vi "Handle Messages.vi"(8 "error in (no error)":errorcluster, 9 "Message Data":variant, 10 "Message":string, 11 "Mock Rig Process In":refnum<class "Mock Error Handler.lvclass">) -> (0 "error out":errorcluster, 3 "Mock Rig Process Out":refnum<class "Mock Error Handler.lvclass">)   [LabVIEW 2020, in "Mock Error Handler.lvclass"]
uses:
  Mock Error Handler.lvclass
  C:/Users/anton/Documents/GitHub/Triarc-Framework/source/Framework/Process/Process.lvclass
  Mock Error Handler.lvclass/Mock Error Handler.ctl
  Framework/Process/Process.lvclass/Process.ctl
  Framework/Process/Process.lvclass
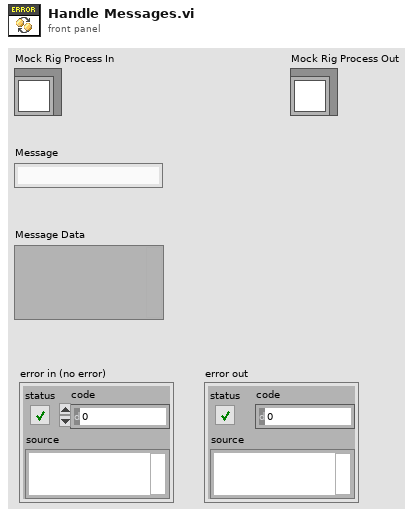
[diagram p1: front panel]
types:
  T1 = cluster{"Message":string, "Message Data":variant}
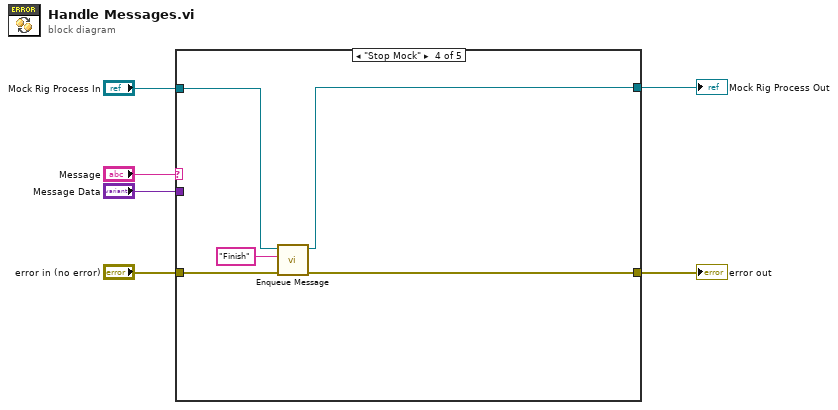
[diagram p0: block diagram]
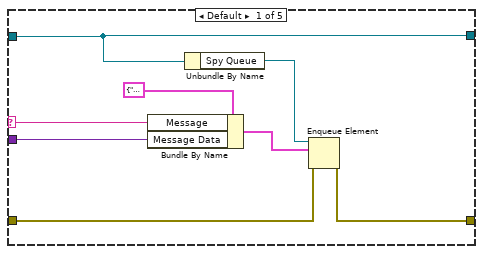
[diagram p2: hidden frame]
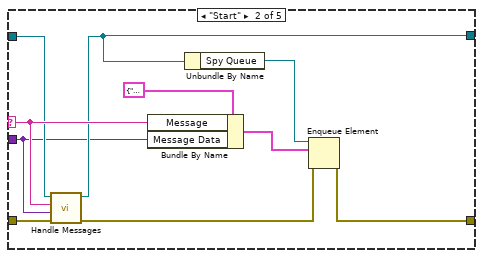
[diagram p3: hidden frame]
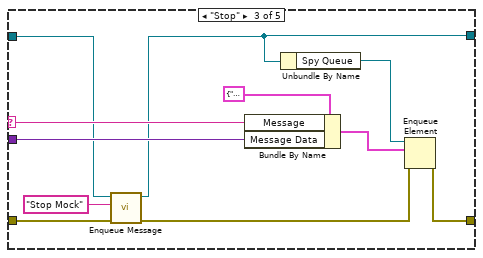
[diagram p4: hidden frame]
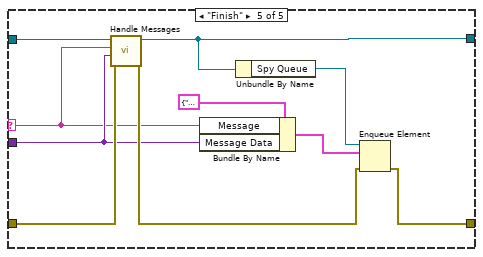
[diagram p5: hidden frame]
diagram:
  n1 = case shown="\"Stop Mock\"" "Message" {
    selector: "Message" -> [w10 w18 w31 _ w41]
    tunnel: [w8 w20 w30 w39 w43] -> w6
    tunnel: [w7 w17 w26 w37 w45] -> w5
    tunnel: "error in (no error)" -> [w9 w21 w27 w38 w49]
    tunnel: "Message Data" -> [w11 w15 w32 _ w42]
    tunnel: "Mock Rig Process In" -> [w7 w16 w25 w36 w50]
    frame Default {
      n2 = Bundle By Name(cluster=T1 {"Message"="", "Message Data"=variant} ("Message Cluster"), "Message"=w10, "Message Data"=w11) -> (w14:T1)
      n3 = Unbundle By Name(w7) -> ("Spy Queue"=w12:refnum<queue>)
      n4 = Enqueue Element(queue=w12, element=w14, error in (no error)=w9) -> (error out=w8:errorcluster)  [unwired: 1 in, 2 out]
    }
    frame "Start" {
      n5 = call-parent "Handle Messages.vi"("error in (no error)"=w21, "Message Data"=w15, "Message"=w18, "Process In"=w16) -> ("error out"=w19:errorcluster, "Process Out"=w17:refnum<class "Mock Error Handler.lvclass">)  [unwired: 6 in]
      n6 = Bundle By Name(cluster=T1 {"Message"="", "Message Data"=variant} ("Message Cluster"), "Message"=w18, "Message Data"=w15) -> (w24:T1)
      n7 = Unbundle By Name(w17) -> ("Spy Queue"=w22:refnum<queue>)
      n8 = Enqueue Element(queue=w22, element=w24, error in (no error)=w19) -> (error out=w20:errorcluster)  [unwired: 1 in, 2 out]
    }
    frame "Stop" {
      n9 = call "Enqueue Message.vi"("error in (no error)"=w27, "Message"="Stop Mock", "Process In"=w25) -> ("error out"=w28:errorcluster, "Process Out"=w26:refnum<class "Mock Error Handler.lvclass">)  [unwired: 7 in]
      n10 = Bundle By Name(cluster=T1 {"Message"="", "Message Data"=variant} ("Message Cluster"), "Message"=w31, "Message Data"=w32) -> (w35:T1)
      n11 = Unbundle By Name(w26) -> ("Spy Queue"=w33:refnum<queue>)
      n12 = Enqueue Element(queue=w33, element=w35, error in (no error)=w28) -> (error out=w30:errorcluster)  [unwired: 1 in, 2 out]
    }
    frame "Stop Mock" {
      n13 = call "Enqueue Message.vi"("error in (no error)"=w38, "Message"="Finish", "Process In"=w36) -> ("error out"=w39:errorcluster, "Process Out"=w37:refnum<class "Mock Error Handler.lvclass">)  [unwired: 7 in]
    }
    frame "Finish" {
      n14 = call-parent "Handle Messages.vi"("error in (no error)"=w49, "Message Data"=w42, "Message"=w41, "Process In"=w50) -> ("error out"=w44:errorcluster, "Process Out"=w45:refnum<class "Mock Error Handler.lvclass">)  [unwired: 6 in]
      n15 = Bundle By Name(cluster=T1 {"Message"="", "Message Data"=variant} ("Message Cluster"), "Message"=w41, "Message Data"=w42) -> (w48:T1)
      n16 = Unbundle By Name(w45) -> ("Spy Queue"=w47:refnum<queue>)
      n17 = Enqueue Element(queue=w47, element=w48, error in (no error)=w44) -> (error out=w43:errorcluster)  [unwired: 1 in, 2 out]
    }
  }
  "error out" <- w6
  "Mock Rig Process Out" <- w5
